vi "Start Configure UI.vi"(8 "error in (no error)":errorcluster, 9 "Container":refnum<vi>, 10 "Project In":refnum<class "Project.lvclass">, 11 "SerializableObject in":refnum<class "SerializableObject.lvclass">) -> (0 "error out":errorcluster, 1 "Configure VI Refnum":refnum<vi>, 3 "SerializableObject out":refnum<class "SerializableObject.lvclass">)   [LabVIEW 2015, in "Editor.lvclass"]
uses:
  Editor.lvclass
  SerializableObject/SerializableObject.lvclass
  Project.lvclass
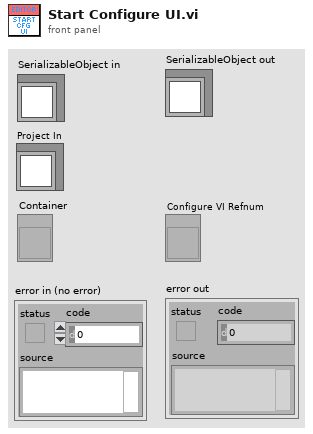
[diagram p1: front panel]
types:
  T1 = enum32{"Invalid", "Standard", "Closed", "Hidden", "Minimized", "Maximized"}
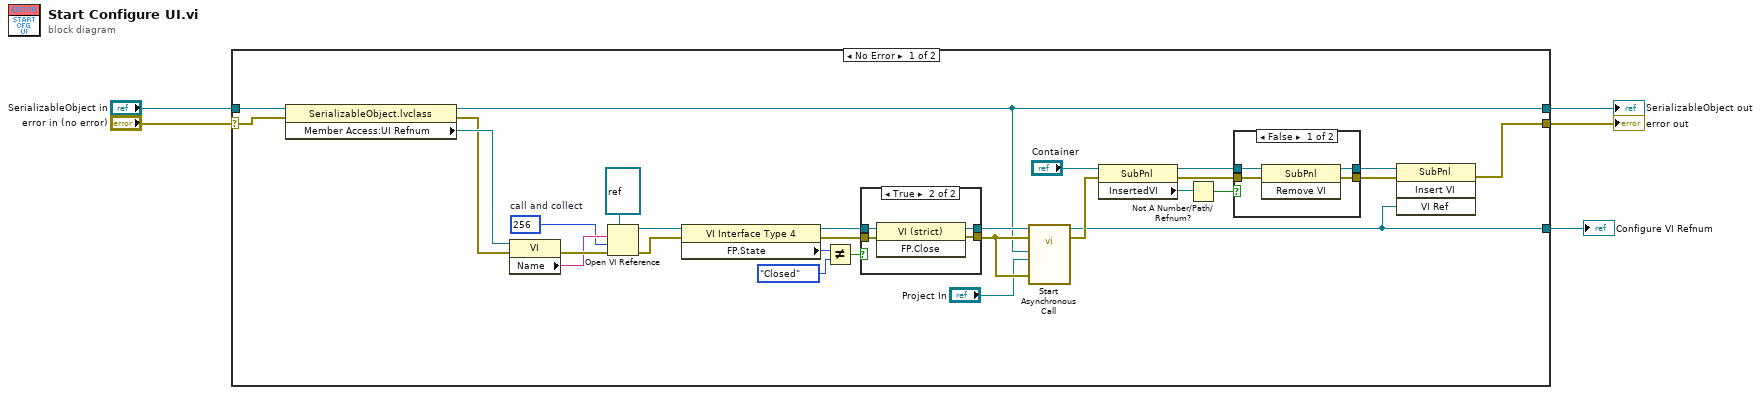
[diagram p0: block diagram]
diagram:
  n1 = case shown="No Error" "error in (no error)" {
    selector: "error in (no error)" -> [w8 w48]
    tunnel: [w23 w48] -> w4
    tunnel: [w10 w47] -> w2
    tunnel: "SerializableObject in" -> [w21 w47]
    tunnel: [w9 _] -> w1
    frame No Error {
      w32 = 256  # call and collect
      n2 = property class="SerializableObject.lvclass"(reference=w21, error in=w8) -> (reference out=w10:refnum<class "SerializableObject.lvclass">, error out=w7:errorcluster, "Member Access:UI Refnum"=w20:refnum<vi>)
      n3 = property class="VI"(reference=w20, error in=w7) -> (error out=w34:errorcluster, "Name"=w33:string)  [unwired: 1 out]
      n4 = Open VI Reference(type specifier VI Refnum (for type only)=refnum<vi> refnum ("VI Refnum"), vi path=w33, options=w32, error in (no error)=w34) -> (vi reference=w19:refnum<vi>, error out=w18:errorcluster)  [unwired: 2 in]
      n5 = property class="VI Interface Type 4"(reference=w19, error in=w18) -> (reference out=w14:refnum<vi>, error out=w13:errorcluster, "FP.State"=w17:T1)
      n6 = Not Equal?(x=w17, y=T1."Closed" ("Front Panel Window:State")) -> (x != y?=w15:bool)
      n7 = case shown="True" w15 {
        tunnel: w14 -> [w42 w46]
        tunnel: w13 -> [w41 w45]
        tunnel: [w42 w44] -> w11
        tunnel: [w41 w43] -> w12
        frame False {
        }
        frame True {
          n8 = invoke class="VI (strict)" method="FP.Close"(reference=w46, error in=w45) -> (reference out=w44:refnum<vi>, error out=w43:errorcluster)  [unwired: 1 in, 1 out]
        }
      }
      n9 = call-by-ref "Start Asynchronous Call"(reference=w11, error in=w12, 8:"error in (no error)"=w12, "Project In"="Project In", "SerializableObject in"=w10) -> (reference out=w9:refnum<vi>, error out=w28:errorcluster)  [unwired: 7 in, 2 out]
      n10 = property class="SubPnl"(reference="Container", error in=w28) -> (reference out=w27:refnum<vi>, error out=w26:errorcluster, "InsertedVI"=w30:refnum<vi>)
      n11 = Not A Number/Path/Refnum?(number/path/refnum=w30) -> (NaN/Path/Refnum?=w29:bool)
      n12 = case shown="False" w29 {
        tunnel: w27 -> [w38 w40]
        tunnel: w26 -> [w37 w39]
        tunnel: [w36 w40] -> w25
        tunnel: [w35 w39] -> w24
        frame False {
          n13 = invoke class="SubPnl" method="Remove VI"(reference=w38, error in=w37) -> (reference out=w36:refnum<vi>, error out=w35:errorcluster)  [unwired: 1 in, 1 out]
        }
        frame True {
        }
      }
      n14 = invoke class="SubPnl" method="Insert VI"(reference=w25, error in=w24, "VI Ref"=w9) -> (error out=w23:errorcluster)  [unwired: 1 in, 3 out]
    }
    frame Error {
    }
  }
  "error out" <- w4
  "SerializableObject out" <- w2
  "Configure VI Refnum" <- w1
